vi "OSICS_Set_Power_SLD.vi"(7 "OSICS slot":i32=1 min=1 max=8 step=1, 8 "error in":errorcluster, 9 "P value":enum16{"Low", "High"}(ring), 10 "Power Unit(False:dBm)":bool, 11 "VISA IN":refnum<visa-resource-name>) -> (0 "error out":errorcluster, 3 "VISA OUT":refnum<visa-resource-name>, 5 "ERR":i32)   [LabVIEW 2014, in "OSICS_LIB.lvlib"]
doc: "This Vi sets the power units and power output value for the OSICS SLED module."
uses:
  OSICS_LIB.lvlib
panel:
  # "Basic Function to set the power units and power output\nfor the OSICS SLED module"
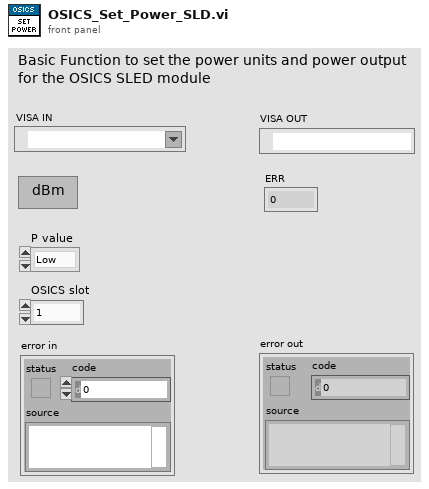
[diagram p1: front panel]
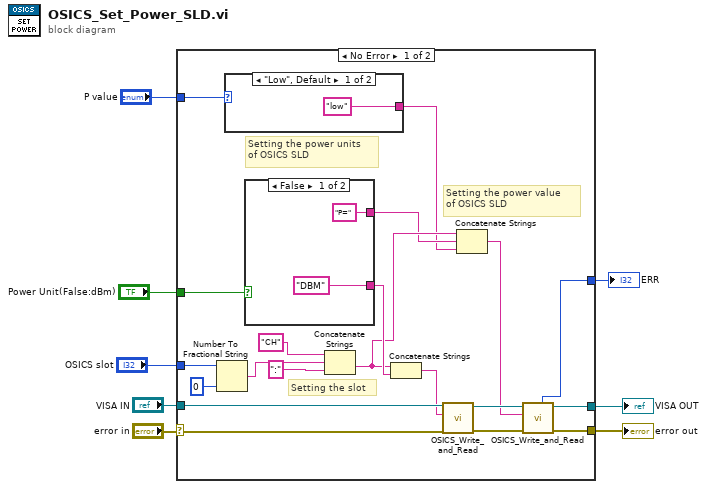
[diagram p0: block diagram]
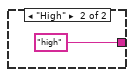
[diagram p2: hidden frame]
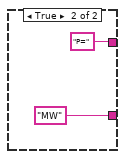
[diagram p3: hidden frame]
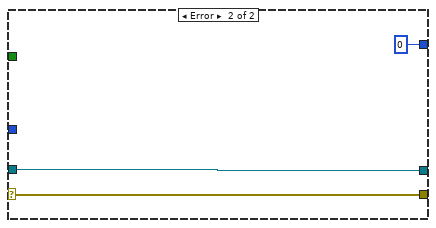
[diagram p4: hidden frame]
diagram:
  n1 = case shown="No Error" "error in" {
    selector: "error in" -> [w22 w36]
    tunnel: "Power Unit(False:dBm)" -> [w28 _]
    tunnel: "VISA IN" -> [w27 w37]
    tunnel: [w24 w37] -> w7
    tunnel: [w23 w36] -> w6
    tunnel: [w9 0 ("ERR")] -> w3
    tunnel: "OSICS slot" -> [w21 _]
    tunnel: "P value" -> [w12 _]
    frame No Error {
      # "Setting the slot"
      # "Setting the power value\nof OSICS SLD"
      # "Setting the power units\nof OSICS SLD"
      n2 = Number To Fractional String(number=w21, precision (6)=i16 0) -> (F-format string=w18:string)  [unwired: 2 in]
      n3 = case shown="\"Low\", Default" w12 {
        tunnel: ["low" "high"] -> w10
        frame "Low", Default {
        }
        frame "High" {
        }
      }
      n4 = case shown="False" w28 {
        tunnel: ["DBM" "MW"] -> w15
        tunnel: ["P=" "P="] -> w13
        frame False {
        }
        frame True {
        }
      }
      n5 = Concatenate Strings("CH" ("string"), w18, ":" ("string")) -> (w14:string)
      n6 = Concatenate Strings(w14, w15) -> (w16:string)
      n7 = call "OSICS_Write_and_Read.vi"("error in (no error)"=w22, "String to Send"=w16, "VISA IN"=w27) -> ("error out"=w25:errorcluster, "VISA OUT"=w26:refnum<visa-resource-name>)  [unwired: 5 in, 2 out]
      n8 = Concatenate Strings(w14, w13, w10) -> (w11:string)
      n9 = call "OSICS_Write_and_Read.vi"("error in (no error)"=w25, "String to Send"=w11, "VISA IN"=w26) -> ("error out"=w23:errorcluster, "VISA OUT"=w24:refnum<visa-resource-name>, "ERR"=w9:i32)  [unwired: 5 in, 1 out]
    }
    frame Error {
    }
  }
  "error out" <- w6
  "VISA OUT" <- w7
  "ERR" <- w3
